vi "水样浓度全局.vi"() -> ()   [LabVIEW 2016, in "质控单元.lvlib"]
panel:
  in  "CODCr加标前水样浓度":dbl
  in  "总氮加标前水样浓度":dbl
  in  "COD加标前水样浓度":dbl
  in  "总磷加标前水样浓度":dbl
  in  "氨氮加标前水样浓度":dbl
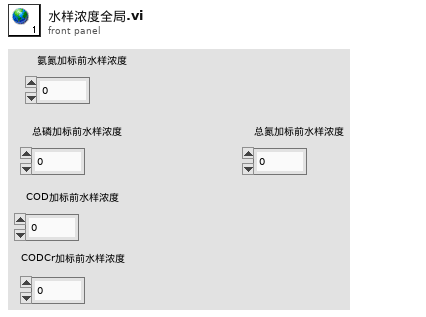
[diagram p1: front panel]
diagram:
